vi "SaveWFMFile.vi"(5 "Settings":T1={"Name of test"="", "Date"=timestamp(0 s since 1904-01-01), "Location"="", "Template"="", "Soundcard"="", "resolution"=32, "Sampling rate"=48000, "Ch1 Gain "=25.0, "Ch2 Gain"=10.0, "Sample time (s)"=0.3, "Pre-trigger (s)"=0.01, "Hammer Threshold"=10.0, "Positions"=12, "Taps/Position"=5, "Set Names"="", "Freq resolution"=10.0, "Hammer cutoff"=0.0, "Mic cutoff"=0.0, "Double bounce "=0.0, "Hammer Cal"=10.0, "dB Offset"=0.0, "Accel Cal"=10.0, "Vibrometer Cal"=0.0, "Mic Cal"=0.0, "Output"=2, "Voltage Cal"=1.0, "Vibrometer Port"="ASRL27::INSTR", "Range"=4, "High Pass"=2, "Bandwidth"=4, "X Range"=[], "Y Range"=[], "dB Spread"=0.0, "Trigger"=0, "Ch_1"=25, "Ch_2"=25, "flip?"=FALSE, "60Hz"=FALSE, "Time offset"=0.0, "Piezo Cal"=1.0, "Default Notes"=""} {"Ch_2" min=1 step=1; "Ch_1" min=1 max=100 step=1; "Trigger" items=["Hammer (force)", "Self-tap", "Spacebar"]; "Bandwidth" items=["1 kHz"=1, "5 kHz"=5, "10 kHz"=10, "25 kHz"=25, "50 kHz"=50, "100 kHz"=100]; "High Pass" items=["Off", "13 Hz", "104 Hz"]; "Range" items=["10 mm/s"=1, "20 mm/s"=2, "50 mm/s"=5, "100 mm/s"=10, "200 mm/s"=20, "500 mm/s"=50, "1 m/s"=100, "2 m/s"=200]; "Output" items=["Accelerometer", "Speed (from acceleration)", "Microphone", "Vibrometer", "Piezo"]; "Voltage Cal" format="%#_13g"; "Ch2 Gain" format="%#_13g"; "Ch1 Gain" format="%#_13g"; "Double bounce" min=0.0; "Mic cutoff" min=0.0 format="%#_4g"; "Hammer cutoff" min=0.0 format="%#_4g"; "Freq resolution" min=0.0; "Pre-trigger (s)" format="%#_13g"; "Date" format="%<%H:%M\n%d/%m/%y>T"; "resolution" items=["16 bit"=16, "24 bit"=24, "32 bit"=32]; "Sampling rate" items=["22050 samp/s"=22050, "44100 samp/s"=44100, "48000 samp/s"=48000]}, 6 "Done? in":bool, 7 "Data":waveform(dbl)[](array[waveform]), 8 "error in (no error)":errorcluster, 9 "New File":string, 10 "Good point?":bool, 11 "Path To Raw Folder":path) -> (0 "error out":errorcluster, 1 "Done? out":bool, 2 "new file path":path, 3 "Canceled":bool)   [LabVIEW 2022 SP3]
uses:
  PreferencesControl.ctl
panel:
  # "Hz"
  # "dB"
  # "dB"
  # "sec"
  # "sec"
  # "mV/Pa"
  # "mV/m/s2"
  # "mV/mm/s"
  # "V/N"
  # "sec"
  # "sec"
  # "mV/N"
  # "a.u."
  # "a.u."
  # "sec"
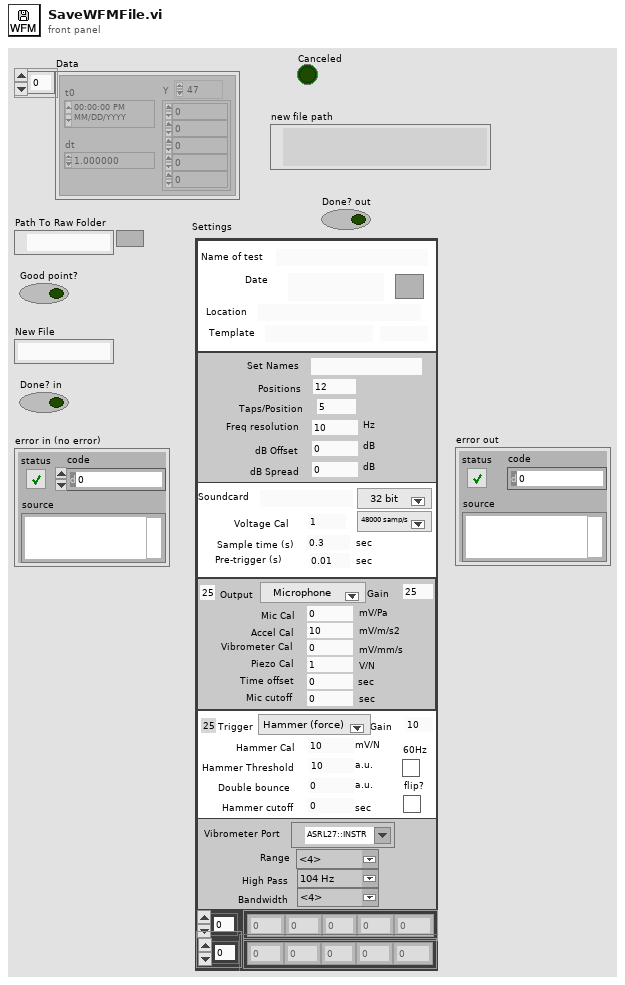
[diagram p1: front panel]
types:
  T1 = typedef "PreferencesControl.ctl" = cluster{"Name of test":string, "Date":timestamp, "Location":string, "Template":string, "Soundcard":string, "resolution":u16, "Sampling rate":u16, "Ch1 Gain ":dbl, "Ch2 Gain":dbl, "Sample time (s)":dbl, "Pre-trigger (s)":dbl, "Hammer Threshold":dbl, "Positions":i16, "Taps/Position":i16, "Set Names":string, "Freq resolution":dbl, "Hammer cutoff":dbl, "Mic cutoff":dbl, "Double bounce ":dbl, "Hammer Cal":dbl, "dB Offset":dbl, "Accel Cal":dbl, "Vibrometer Cal":dbl, "Mic Cal":dbl, "Output":u16, "Voltage Cal":dbl, "Vibrometer Port":refnum<visa-resource-name>, "Range":u16, "High Pass":u16, "Bandwidth":u16, "X Range":cluster{"Minimum":dbl, "Maximum":dbl, "Increment":dbl, "Minor Increment":dbl, "Start":dbl}[], "Y Range":cluster{"Minimum":dbl, "Maximum":dbl, "Increment":dbl, "Minor Increment":dbl, "Start":dbl}[], "dB Spread":dbl, "Trigger":u16, "Ch_1":u8, "Ch_2":u8, "flip?":bool, "60Hz":bool, "Time offset":dbl, "Piezo Cal":dbl, "Default Notes":string}
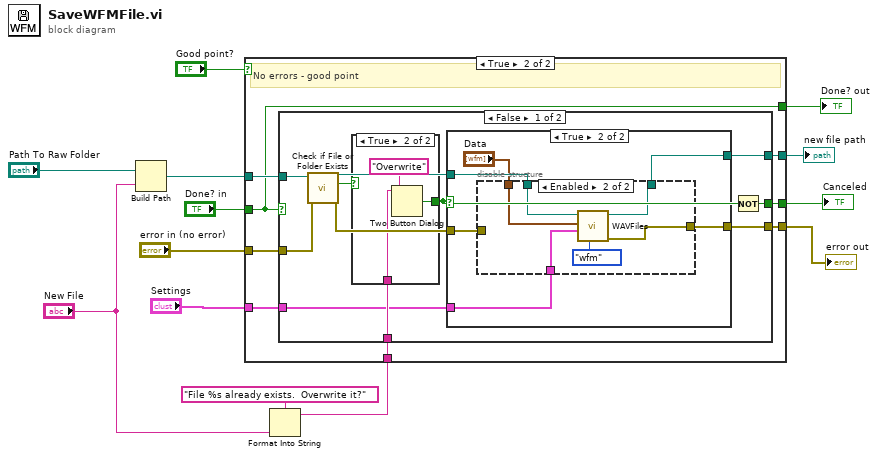
[diagram p0: block diagram]
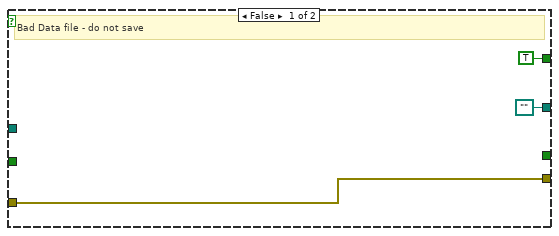
[diagram p2: hidden frame]
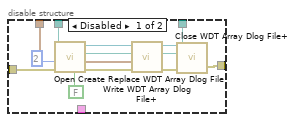
[diagram p4: hidden frame]
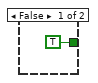
[diagram p5: hidden frame]
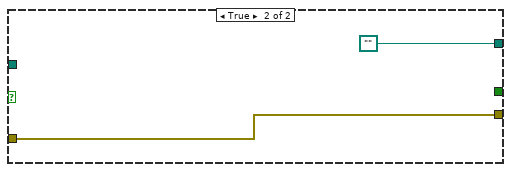
[diagram p6: hidden frame]
diagram:
  n1 = Build Path(base path="Path To Raw Folder", name or relative path="New File") -> (appended path=w11:path)
  n2 = Format Into String(format string="File %s already exists.  Overwrite it?" ("message"), "New File") -> (resulting string=w6:string)  [unwired: 2 in, 1 out]
  n3 = case shown="True" "Good point?" {
    tunnel: "error in (no error)" -> [w15 w24]
    tunnel: w6 -> [_ w23]
    tunnel: [path "" ("new file path") w22] -> w7
    tunnel: [w15 w21] -> w9
    tunnel: "Done? in" -> [_ w19]
    tunnel: w11 -> [_ w20]
    tunnel: [TRUE ("Done?") w19] -> w13
    tunnel: [_ w18] -> w2
    tunnel: "Settings" -> [_ w17]
    frame False {
      # "Bad Data file - do not save"
    }
    frame True {
      # "No errors - good point"
      n4 = case shown="False" w19 {
        tunnel: w24 -> [w32 w65]
        tunnel: [w35 w65] -> w21
        tunnel: w20 -> [w33 _]
        tunnel: [w34 path "" ("new file path")] -> w22
        tunnel: w23 -> [w28 _]
        tunnel: [w26 _] -> w18
        tunnel: w17 -> [w25 _]
        frame False {
          n5 = call <vilib>:"Check if File or Folder Exists.vi"("error in (no error)"=w32, "path"=w33) -> ("error out"=w31:errorcluster, "file or folder exists?"=w30:bool, "dup path"=w29:path)  [unwired: 7 in]
          n6 = case shown="True" w30 {
            tunnel: [TRUE ("true") w63] -> w27
            tunnel: w28 -> [_ w62]
            frame False {
            }
            frame True {
              n7 = Two Button Dialog(message=w62, 2:"Overwrite" ("T button name (\"OK\")")) -> (T button?=w63:bool)  [unwired: 1 in]
            }
          }
          n8 = case shown="True" w27 {
            tunnel: [w37 w40] -> w35
            tunnel: [w36 w41] -> w34
            tunnel: w31 -> [w37 w43]
            tunnel: w29 -> [w36 w42]
            tunnel: w25 -> [_ w38]
            frame False {
            }
            frame True {
              n9 = disable-structure shown="Enabled" {
                disable-tunnel: w43 -> [w48 _]
                disable-tunnel: w42 -> [w47 w56]
                disable-tunnel: [w46 w56] -> w41
                disable-tunnel: [w45 w57] -> w40
                disable-tunnel: "Data" -> [w44 w58]
                disable-tunnel: w38 -> [_ w55]
                frame Disabled {
                  n10 = call <vilib>:"Open Create Replace WDT Array Dlog File.vi"("advisory dialog? (display:T)"=FALSE, "error in (not an error)"=w48, "function (open:0)"=i16 2 ("create or replace"), "file path"=w47) -> ("error out"=w51:errorcluster, "new file path"=w46:path, "refnum"=w52:refnum<k1>)  [unwired: 4 in, 1 out]
                  n11 = call <vilib>:"Write WDT Array Dlog File+.vi"("error in (no error)"=w51, "Array"=w44, "refnum"=w52) -> ("error out"=w54:errorcluster, "refnum"=w53:refnum<k1>)  [unwired: 6 in, 1 out]
                  n12 = call <vilib>:"Close WDT Array Dlog File+.vi"("error in (no error)"=w54, "refnum"=w53) -> ("error out"=w45:errorcluster)  [unwired: 3 in, 2 out]
                }
                frame Enabled {
                  n13 = call "WAVFiles.vi"("Task"=enum16{"Read", "Write", "wfm"}."wfm", "Settings"=w55, "Wfm data"=w58, "WAV File"=w56) -> ("error out"=w57:errorcluster)  [unwired: 4 in, 3 out]
                }
              }
            }
          }
          n14 = Not(x=w27) -> (.not. x?=w26:bool)
        }
        frame True {
        }
      }
    }
  }
  "Done? out" <- w13
  "error out" <- w9
  "new file path" <- w7
  "Canceled" <- w2
